vi "wait.vi"(0 "HGF_Notifier":refnum<class "HGF_Notifier.lvclass">, 3 "msTimeout (-1)":i32=-1, 5 "error in (no error)":errorcluster, 9 "ignore previous (F)":bool) -> (14 "dup HGF_Notifier":refnum<class "HGF_Notifier.lvclass">, 16 "Object":refnum<class>, 17 "timed out":bool, 19 "error out":errorcluster)   [LabVIEW 2014, in "HGF_BaseClasses.lvlib" / "HGF_Notifier.lvclass"]
doc: "Use this VI to wait on events. It returns the default object in case of timeout.\n\n<b>Hint:</b> This is a shared reentrant VI."
uses:
  HGF_Notifier.lvclass
  HGF_Event/HGF_Event.lvclass
  HGF_Auxiliary/HGF_Auxiliary.lvlib
  HGF_Auxiliary/Severity.ctl
  HGF_Auxiliary/ErrorCode.ctl
  HGF_Timing/HGF_Timing.lvclass
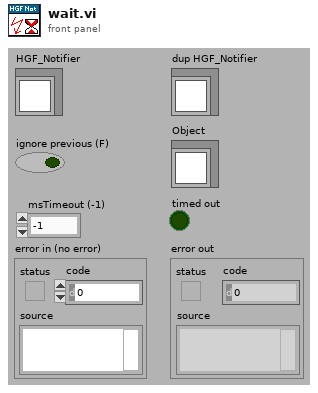
[diagram p1: front panel]
types:
  T1 = typedef "HGF_Auxiliary.lvlib/ErrorCode.ctl" = enum32{"No error", "Function not supported.", "This VI is for friends only.", "Reference object aready exisits.", "Parameter out of range.", "Not a rendezvous.", "Invalid notifier reference.", "Invalid queue reference.", "Self-Test not supported.", "Reset not supported.", "IDN query not supported.", "Error query not supported.", "Incorrect addressee.", "Object already exists.", "No class name specified", "Driver not supported", "Attribute is not writable"}
  T2 = typedef "HGF_Auxiliary.lvlib/Severity.ctl" = enum16{"Info", "Warning", "Fault", "Error", "Fatal"}
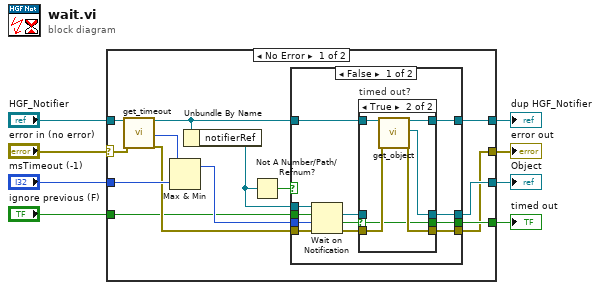
[diagram p0: block diagram]
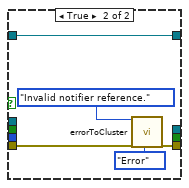
[diagram p3: hidden frame]
diagram:
  n1 = case shown="No Error" "error in (no error)" {
    selector: "error in (no error)" -> [w19 w50]
    tunnel: "HGF_Notifier" -> [w22 w51]
    tunnel: [w9 w51] -> w1
    tunnel: [w21 _] -> w3
    tunnel: [w20 _] -> w2
    tunnel: "msTimeout (-1)" -> [w16 _]
    tunnel: "ignore previous (F)" -> [w14 _]
    tunnel: [w13 w50] -> w4
    frame No Error {
      n2 = call "get_timeout.vi"("HGF_Event.lvclass in"=w22, "error in (no error)"=w19) -> ("HGF_Event.lvclass out"=w10:refnum<class "HGF_Notifier.lvclass">, "timeout"=w18:i32, "error out"=w15:errorcluster)  [unwired: 15 out]
      n3 = Max & Min(x=w18, y=w16) -> (max(x,y)=w17:i32)  [unwired: 1 out]
      n4 = Unbundle By Name(w10) -> ("notifierRef"=w11:refnum<notifier>)
      n5 = Not A Number/Path/Refnum?(number/path/refnum=w11) -> (NaN/Path/Refnum?=w12:bool)
      n6 = case shown="False" w12 {
        tunnel: [w25 _] -> w21
        tunnel: [w24 _] -> w20
        tunnel: w17 -> [w34 _]
        tunnel: w15 -> [w33 w48]
        tunnel: w11 -> [w32 _]
        tunnel: w14 -> [w31 _]
        tunnel: [w27 w49] -> w13
        tunnel: w10 -> [w30 w45]
        tunnel: [w29 w45] -> w9
        frame False {
          n7 = Wait on Notification(notifier=w32, ignore previous (F)=w31, timeout in ms (-1)=w34, error in (no error)=w33) -> (notification=w23:refnum<class>, timed out?=w26:bool, error out=w28:errorcluster)  [unwired: 1 out]
          n8 = case "timed out?" shown="True" w26 {
            selector: w26 -> [w38 w40]
            tunnel: w30 -> [w36 w44]
            tunnel: [w36 w43] -> w29
            tunnel: w28 -> [w37 w42]
            tunnel: [w37 w41] -> w27
            tunnel: [w38 w40] -> w25
            tunnel: [w35 w39] -> w24
            tunnel: w23 -> [w35 _]
            frame False {
            }
            frame True {
              n9 = call "get_object.vi"("HGF_Timing.lvclass"=w44, "error in (no error)"=w42) -> ("dup HGF_Timing"=w43:refnum<class "HGF_Notifier.lvclass">, "object"=w39:refnum<class>, "error out"=w41:errorcluster)  [unwired: 15 out]
            }
          }
        }
        frame True {
          n10 = call "errorToCluster.vi"("error code"=ErrorCode."Invalid notifier reference." ("HGF_Error"), "error in (no error)"=w48, "severity (Error)"=Severity."Error") -> ("error out"=w49:errorcluster)  [unwired: 2 in, 14 out]
        }
      }
    }
    frame Error {
    }
  }
  "error out" <- w4
  "dup HGF_Notifier" <- w1
  "timed out" <- w3
  "Object" <- w2
